vi "GetPTError.vi"(6 "mail info":T1={"host"="smtp-mail.outlook.com", "port"=587, "username"="", "password"="", "From"="", "to"="", "subject"=""}, 7 "params":T2(array[cluster]), 8 "normal? (in, old)":bool[](array[boolean]), 9 "PT values":dbl[](array[numeric])) -> (0 "emailed number":u32, 1 "last emailed msg":string, 2 "normal? (out, new)":bool[](array[boolean]), 3 "overlevel msg":string)   [LabVIEW 2017]
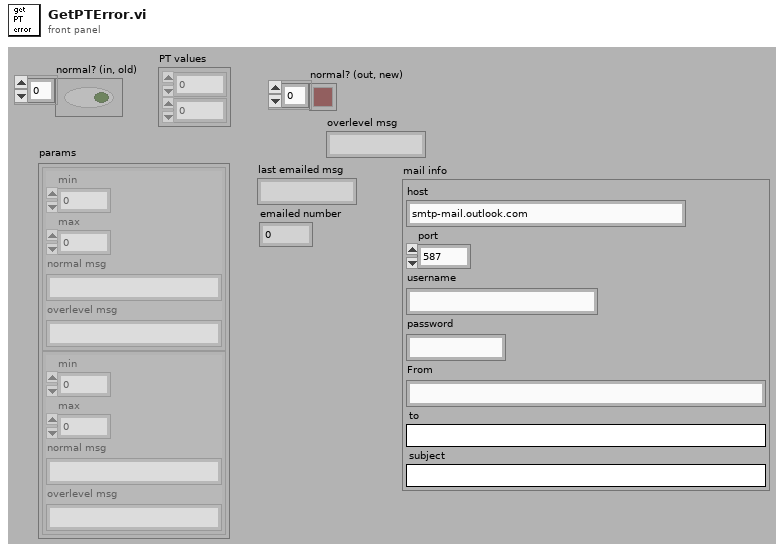
[diagram p1: front panel]
types:
  T1 = cluster{"host":string, "port":i32, "username":string, "password":string, "From":string, "to":string, "subject":string}
  T2 = cluster{"min":dbl, "max":dbl, "normal msg":string, "overlevel msg":string}[]
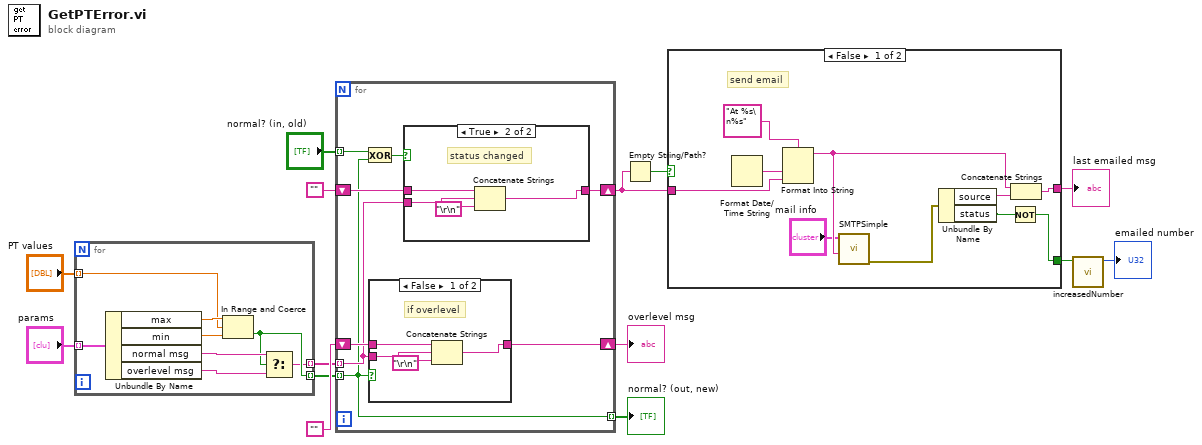
[diagram p0: block diagram]
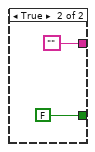
[diagram p2: hidden frame]
diagram:
  n1 = for {
    tunnel: "params" -> [w22] mode=indexing
    tunnel: "PT values" -> [w19] mode=indexing
    tunnel: [w16] -> w4 mode=indexing
    tunnel: [w15] -> w3 mode=indexing
    n2 = Unbundle By Name(w22) -> ("max"=w21:dbl, "min"=w20:dbl, "normal msg"=w18:string, "overlevel msg"=w17:string)
    n3 = In Range and Coerce(upper limit=w21, x=w19, lower limit=w20) -> (In Range?=w16:bool)  [unwired: 1 out]
    n4 = Select(t=w18, s=w16, f=w17) -> (s? t:f=w15:string)
  }
  n5 = for {
    tunnel: "normal? (in, old)" -> [w30] mode=indexing
    tunnel: w4 -> [w23] mode=indexing
    tunnel: w3 -> [w24] mode=indexing
    shift-right: [w28] -> w12
    shift-left: "" -> [w27]
    shift-right: [w25] -> w9
    shift-left: "" -> [w26]
    tunnel: [w23] -> w7 mode=indexing
    n6 = Exclusive Or(1:w23, 2:w30) -> (0:w29:bool)
    n7 = case shown="False" w23 {
      tunnel: w26 -> [w34 w35]
      tunnel: [w33 w35] -> w25
      tunnel: w24 -> [w32 _]
      frame False {
        # "if overlevel"
        n8 = Concatenate Strings(w34, w32, "\r\n") -> (w33:string)
      }
      frame True {
        # "normal"
      }
    }
    n9 = case shown="True" w29 {
      tunnel: w24 -> [_ w38]
      tunnel: [w36 w40] -> w28
      tunnel: w27 -> [w36 w39]
      frame False {
        # "status unchanged"
      }
      frame True {
        # "status changed"
        n10 = Concatenate Strings(w39, w38, "\r\n") -> (w40:string)
      }
    }
  }
  "normal? (out, new)" <- w7
  "overlevel msg" <- w9
  n11 = Empty String/Path?(string/path=w12) -> (empty?=w11:bool)
  n12 = case shown="False" w11 {
    tunnel: w12 -> [w48 _]
    tunnel: [w44 ""] -> w8
    tunnel: [w42 FALSE] -> w1
    frame False {
      # "send email"
      n13 = Format Date/Time String() -> (date/time string=w49:string)  [unwired: 3 out]
      n14 = Format Into String(format string="At %s\n%s" ("格式字符串"), w49, w48) -> (resulting string=w46:string)  [unwired: 2 in, 1 out]
      n15 = call "SMTPSimple.vi"("body"=w46, "mail info"="mail info") -> ("error out"=w47:errorcluster)  [unwired: 1 in, 8 out]
      n16 = Unbundle By Name(w47) -> ("source"=w45:string, "status"=w43:bool)
      n17 = Not(x=w43) -> (.not. x?=w42:bool)
      n18 = Concatenate Strings(w46, w45) -> (w44:string)
    }
    frame True {
    }
  }
  "last emailed msg" <- w8
  n19 = call "increasedNumber.vi"("increase?"=w1) -> ("increased n"=→"emailed number":u32)  [unwired: 10 out]
